vi "2020_day10.vi"() -> ()   [LabVIEW 2021]
uses:
  <userlib>/_OpenG.lib/array/array.llb/Sort 1D Array (I32)__ogtk.vi
  <userlib>/_OpenG.lib/array/array.llb/Search 1D Array (I32)__ogtk.vi
  <vilib>/gmath/NI_Gmath.lvlib
panel:
  out "product":i32
  out "Number of consecutive 1":i32[](array[numeric])
  out "x-y":i32[](array[numeric])
  out "x/y":dbl
  out "Task 1":i32
  in  "Switch":bool caption="Ex. Data  vs.  User Data"
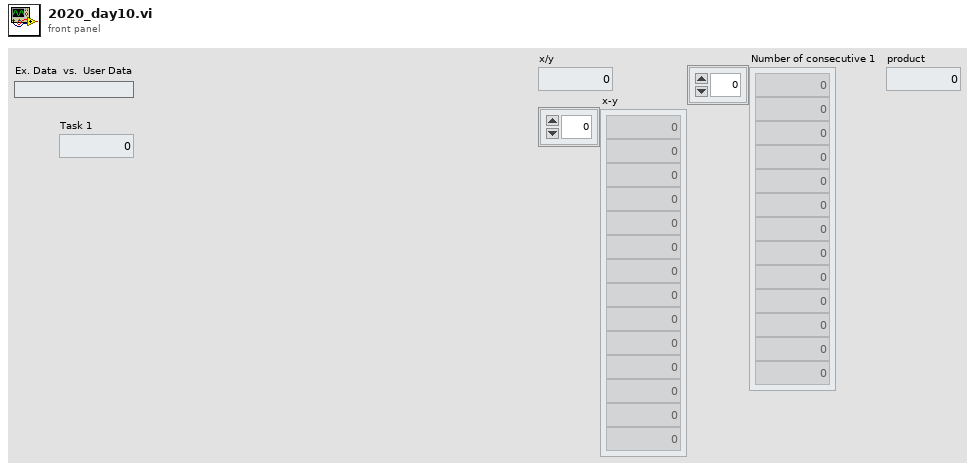
[diagram p1: front panel]
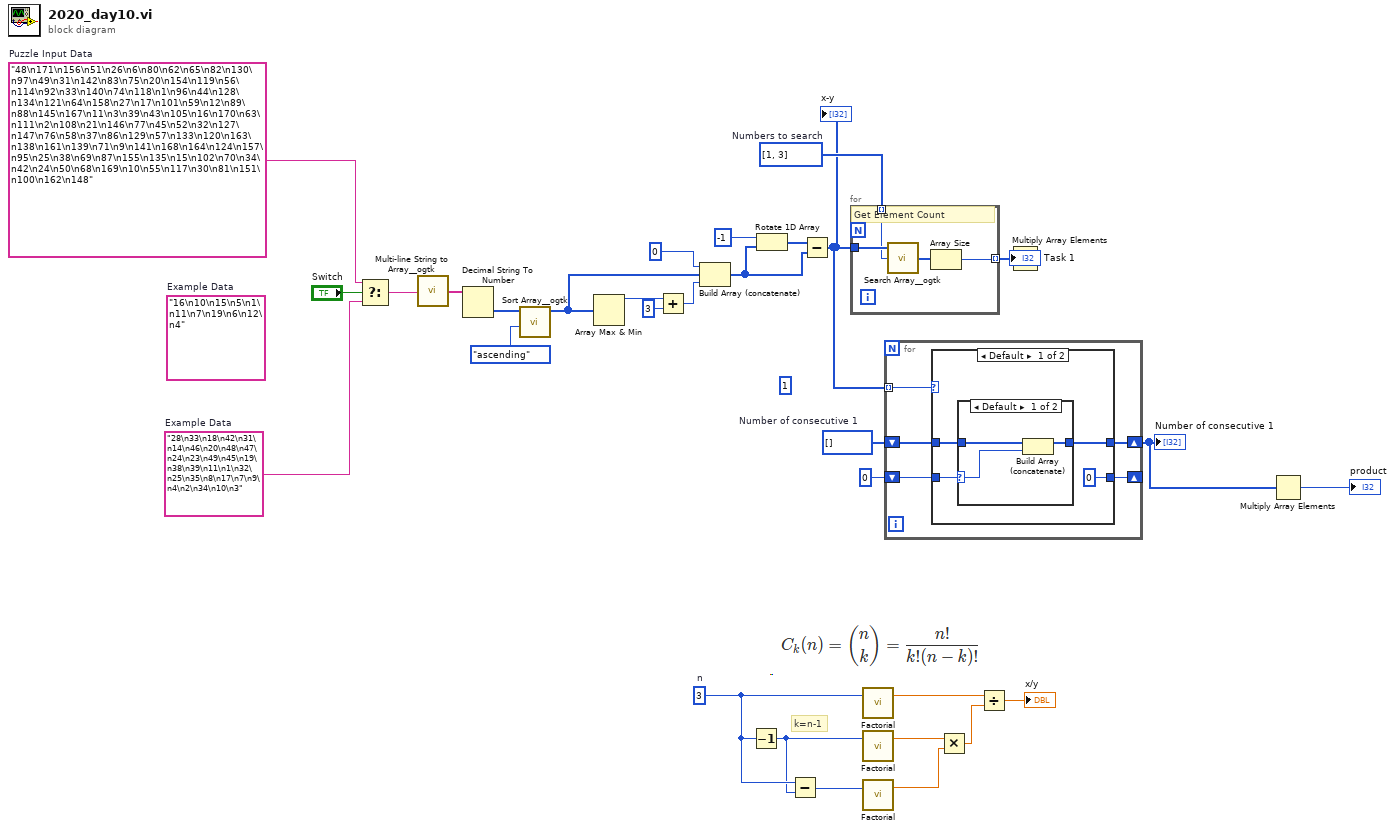
[diagram p0: block diagram]
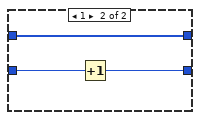
[diagram p3: hidden frame]
diagram:
  w1 = "28\n33\n18\n42\n31\n14\n46\n20\n48\n47\n24\n23\n49\n45\n19\n38\n39\n11\n1\n32\n25\n35\n8\n17\n7\n9\n4\n2\n34\n10\n3"  # Example Data
  w5 = i32[] []  # Number of consecutive 1
  (unwired) 1 ("n")
  w10 = 3  # n
  w18 = i32[] [1, 3]  # Numbers to search
  w30 = "48\n171\n156\n51\n26\n6\n80\n62\n65\n82\n130\n97\n49\n31\n142\n83\n75\n20\n154\n119\n56\n114\n92\n33\n140\n74\n118\n1\n96\n44\n128\n134\n121\n64\n158\n27\n17\n101\n59\n12\n89\n88\n145\n167\n11\n3\n39\n43\n105\n16\n170\n63\n111\n2\n108\n21\n146\n77\n45\n52\n32\n127\n147\n76\n58\n37\n86\n129\n57\n133\n120\n163\n138\n161\n139\n71\n9\n141\n168\n164\n124\n157\n95\n25\n38\n69\n87\n155\n135\n15\n102\n70\n34\n42\n24\n50\n68\n169\n10\n55\n117\n30\n81\n151\n100\n162\n148"  # Puzzle Input Data
  (unwired) "16\n10\n15\n5\n1\n11\n7\n19\n6\n12\n4"  # Example Data
  # "k=n-1"
  n1 = Select(t=w30, s="Switch", f=w1) -> (s? t:f=w29:string)
  n2 = call <userlib>:"Multi-line String to Array__ogtk.vi"("string"=w29) -> ("lines"=w28:string[])
  n3 = Decimal String To Number(string=w28) -> (number=w26:i32[])  [unwired: 2 in, 1 out]
  n4 = call-poly <userlib>:"Sort Array__ogtk.vi"("Order"=enum16{"ascending", "descending"}."ascending", "Array in"=w26) -> ("Sorted Array out"=w23:i32[])  [unwired: 8 in, 1 out]
  n5 = Array Max & Min(array=w23) -> (max value=w22:i32)  [unwired: 3 out]
  n6 = Add(x=w22, y=3) -> (x+y=w21:i32)
  n7 = Build Array (concatenate)(0 ("y"), w23, w21) -> (w17:i32[])
  n8 = Decrement(x=w10) -> (x-1=w9:i32)
  n9 = Rotate 1D Array(1:w17, 2:-1 ("n")) -> (0:w24:i32[])
  n10 = Subtract(x=w10, y=w9) -> (x-y=w11:i32)
  n11 = Subtract(x=w24, y=w17) -> (x-y=w4:i32[])
  "x-y" <- w4
  n12 = for {
    tunnel: w4 -> [w35]
    tunnel: [w34] -> w16 mode=indexing
    tunnel: w18 -> [w33] mode=indexing
    # "Get Element Count"
    n13 = call-poly <userlib>:"Search Array__ogtk.vi"("Array"=w35, "Element Data"=w33) -> ("Indices of Elements"=w32:i32[])  [unwired: 7 in]
    n14 = Array Size(array=w32) -> (size(s)=w34:i32)
  }
  n15 = call <vilib>:"Factorial.vi"("n"=w10) -> ("n!"=w14:dbl)  [unwired: 2 in]
  n16 = call <vilib>:"Factorial.vi"("n"=w9) -> ("n!"=w13:dbl)  [unwired: 2 in]
  n17 = call <vilib>:"Factorial.vi"("n"=w11) -> ("n!"=w8:dbl)  [unwired: 2 in]
  n18 = for {
    shift-right: [w39] -> _
    shift-left: 0 ("n") -> [w40]
    shift-right: [w38] -> w3
    shift-left: w5 -> [w37]
    tunnel: w4 -> [w36] mode=indexing
    n19 = case shown="Default" w36 {
      tunnel: w40 -> [w41 w51]
      tunnel: [0 ("n") w50] -> w39
      tunnel: w37 -> [w43 w49]
      tunnel: [w42 w49] -> w38
      frame Default {
        n20 = case shown="Default" w41 {
          selector: w41 -> [w45 _]
          tunnel: w43 -> [w47 w48]
          tunnel: [w46 w48] -> w42
          frame Default {
            n21 = Build Array (concatenate)(w47, w45) -> (w46:i32[])
          }
          frame 0 {
          }
        }
      }
      frame 1 {
        n22 = Increment(x=w51) -> (x+1=w50:i32)
      }
    }
  }
  "Number of consecutive 1" <- w3
  n23 = Multiply(x=w13, y=w8) -> (x*y=w12:dbl)
  n24 = Divide(x=w14, y=w12) -> (x/y=→"x/y":dbl)
  n25 = Multiply Array Elements(1:w16) -> (0:→"Task 1":i32)
  n26 = Multiply Array Elements(1:w3) -> (0:→"product":i32)
